vi "Build Create.vi"(8 "error in (no error)":errorcluster, 9 "tableName":string, 10 "DynamicParameters in":refnum<class "DynamicParameters.lvclass">, 11 "PostgresqlConnection in":refnum<class "DBC.lvclass">) -> (0 "error out":errorcluster, 1 "LastIdentityQuery":string, 2 "InsertStatement":string, 3 "PostgresqlConnection out":refnum<class "DBC.lvclass">)   [LabVIEW 2020, in "ORM_DBC_Npgsql.lvlib" / "DBC.lvclass"]
uses:
  DBC.lvclass
  <vilib>/Viviota/shared/ORM.lvlibp/ORM/DynamicParameters/DynamicParameters.lvclass
  <vilib>/Viviota/shared/ORM.lvlibp/ORM/DynamicParameters/Read AutoKey.vi
  <vilib>/Viviota/shared/ORM_DBC_dotNet.lvlibp/dbcDotNet/ORM_DBC_dotNet.lvclass
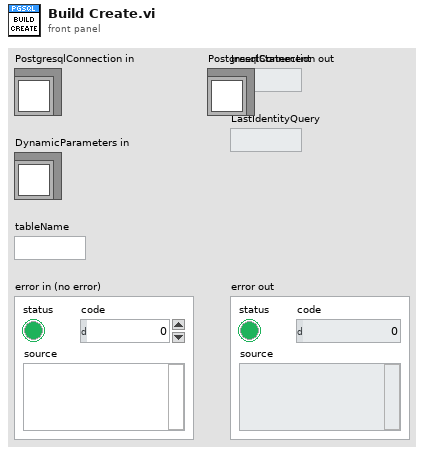
[diagram p1: front panel]
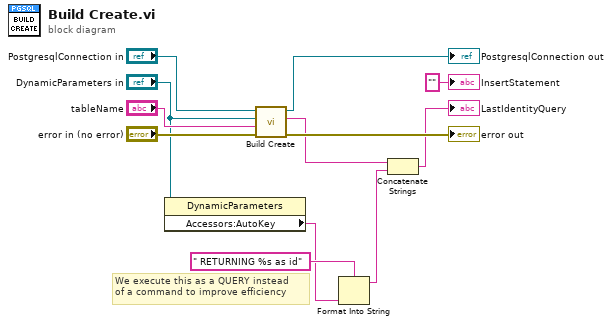
[diagram p0: block diagram]
diagram:
  # "We execute this as a QUERY instead\nof a command to improve efficiency"
  n1 = property class="DynamicParameters"(reference="DynamicParameters in") -> ("Accessors:AutoKey"=w4:string)  [unwired: 1 in, 2 out]
  n2 = call-parent "Build Create.vi"("error in (no error)"="error in (no error)", "tableName"="tableName", "DynamicParameters in"="DynamicParameters in", "DbConnection in"="PostgresqlConnection in") -> ("error out"=→"error out":errorcluster, "InsertStatement"=w7:string, "DbConnection out"=→"PostgresqlConnection out":refnum<class "DBC.lvclass">)  [unwired: 4 in, 1 out]
  n3 = Format Into String(format string=" RETURNING %s as id" ("string"), w4) -> (resulting string=w3:string)  [unwired: 2 in, 1 out]
  n4 = Concatenate Strings(w7, w3) -> (→"LastIdentityQuery":string)
  "InsertStatement" <- "" ("InsertStatement")
